vi "Calculator.vi"() -> ()   [LabVIEW 2018]
panel:
  in  "Ring":u16(ring) items=["*", "+", "-", "/"]
  in  "Число №2":dbl
  in  "Число №1":dbl
  out "Результат":dbl
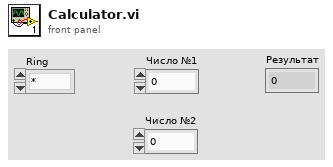
[diagram p1: front panel]
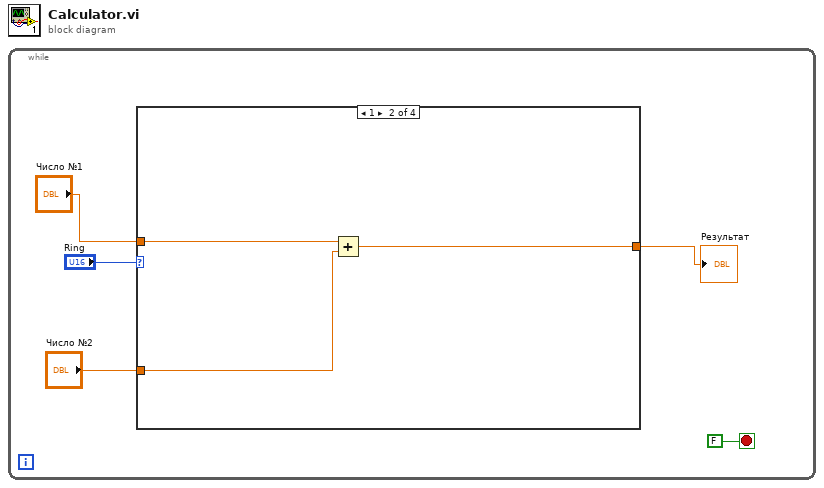
[diagram p0: block diagram]
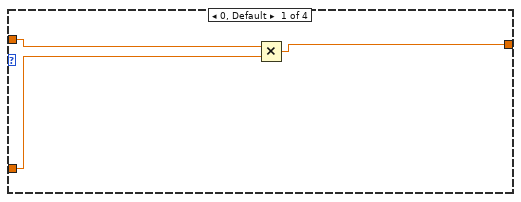
[diagram p2: hidden frame]
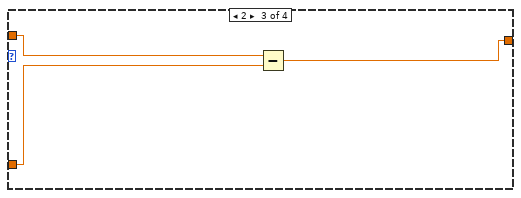
[diagram p3: hidden frame]
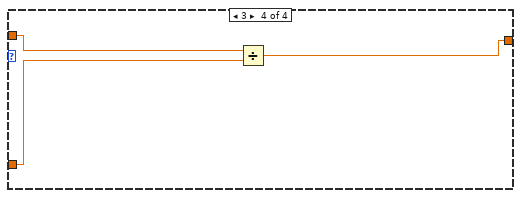
[diagram p4: hidden frame]
diagram:
  n1 = while {
    stop <- FALSE stop-if-true
    n2 = case shown="1" "Ring" {
      tunnel: [w8 w9 w14 w15] -> w5
      tunnel: "Число №1" -> [w7 w11 w13 w17]
      tunnel: "Число №2" -> [w6 w10 w12 w16]
      frame 0, Default {
        n3 = Multiply(x=w7, y=w6) -> (x*y=w8:dbl)
      }
      frame 1 {
        n4 = Add(x=w11, y=w10) -> (x+y=w9:dbl)
      }
      frame 2 {
        n5 = Subtract(x=w13, y=w12) -> (x-y=w14:dbl)
      }
      frame 3 {
        n6 = Divide(x=w17, y=w16) -> (x/y=w15:dbl)
      }
    }
    "Результат" <- w5
  }
